vi "About.vi"   [LabVIEW 2018]
panel:
  # "广东和氏工业技术集团股份有限公司\nGUANGDONG HESH INDUSTRY TECHNOLOGY GROUP CO.,LTD."
  # "广东和氏工业技术集团股份有限公司（股票简称：和氏技术，股票代码:832281）始创于2004年，是国内领先的集研发、生产及销售为一体的高端智能装备解决方案供应商，拥有多项专利及软件著作权，具有完全自主知识产权，是国家高新技术企业。公司于2015年4月在新三板挂牌上市。\n    和氏技术的产品包括高精智能去毛刺抛光机、智能在线质量检测装配线、工业机器人等，广泛应用于汽车、空调、制冷压缩机、电子、家用电器、机械制造、金属材料加工、军工、航空等行业。\n    经过十多年的积累与创新，领先的技术和优良的品质，使得和氏技术的产品及服务大大提升了客户的市场竞争力，获得了客户的广泛青睐和赞誉。\n    地    址：广东省珠海市金湾区联港工业区虹晖五路12号\n    联系电话：0756-3878373 \n    邮    箱：hesh@zh-heshi.com\n\n    合肥和氏自动化技术有限公司是珠海和氏自动化设备有限公司全资公司。合肥和氏秉承着珠海和氏的方针和宗旨，致力于先进自动化装备的研发、制造和服务，公司拥有高素质的研发队伍、先进的制造设备、以及高品质的制造水平，注重团队精神的建设。\n    地    址：安徽省合肥市高新区科学大道与红枫路交口（中瑞大厦A座1306室）\n    联系方式：0551-65302130"
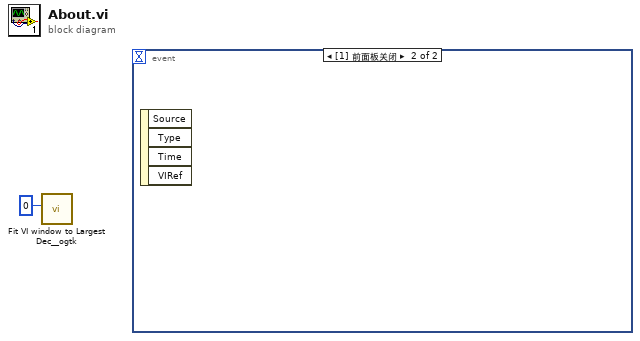
[diagram p0: block diagram]
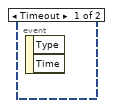
[diagram p2: hidden frame]
diagram:
  n1 = call <userlib>:"Fit VI window to Largest Dec__ogtk.vi"("border spacing (2 px)"=0) -> ()  [unwired: 5 in, 2 out]
  n2 = event shown="[1] 前面板关闭" {
    selector: _ -> [_ _]
    dyn-events: _ -> [_ _]
    timeout: _ -> [_ _]
    event Timeout {
      n3 = event-data() -> ()  [unwired: 1 in, 2 out]
    }
    event Panel Close {
      n4 = event-data() -> ()  [unwired: 1 in, 4 out]
    }
  }
